vi "Flancos_2.vi"() -> ()   [LabVIEW 2017]
panel:
  out "Conteo 4":bool
  out "Conteo 3":bool
  out "Conteo 2":bool
  in  "Alarma":bool
  in  "Alarma 2":bool
  in  "Alarma 3":bool
  in  "Alarma 4":bool
  out "Conteo":bool
  in  "Seleccion":bool
  out "Waveform Chart":dbl(graph)
  out "Falling 4":dbl
  out "Rise 4":dbl
  out "Falling 3":dbl
  out "Rise 3":dbl
  out "Falling 2":dbl
  out "Rise 2":dbl
  out "Falling":dbl
  out "Rise":dbl
  in  "stop":bool
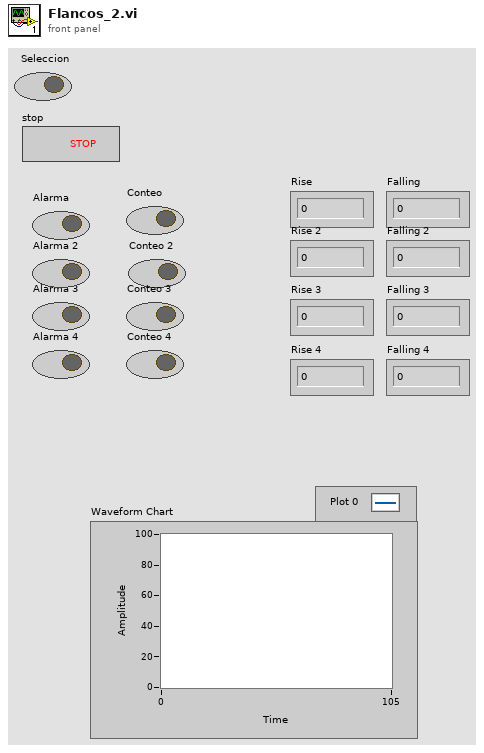
[diagram p1: front panel]
types:
  T1 = cluster{"Cont":i32, "Cont2":i32, "Cont3":i32, "Cont4":i32, "Bajada":i32, "Bajada 2":i32, "Bajada 3":i32, "Bajada 4":i32}
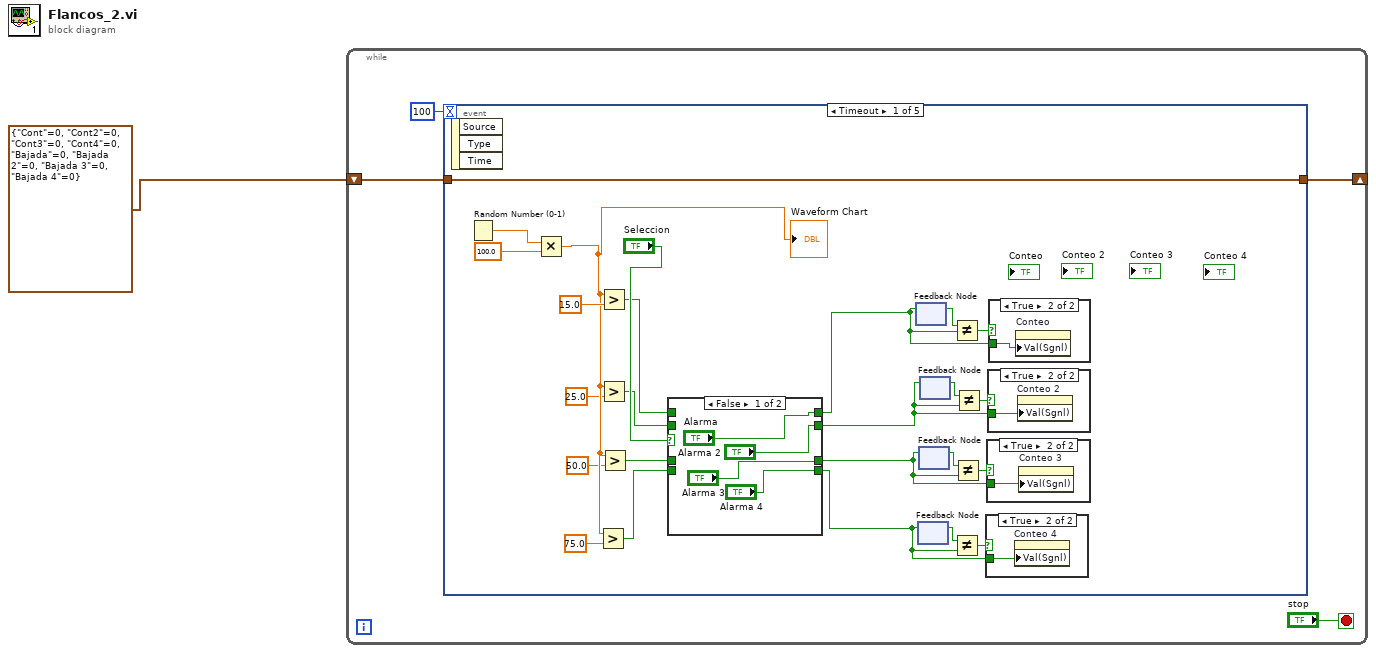
[diagram p0: block diagram]
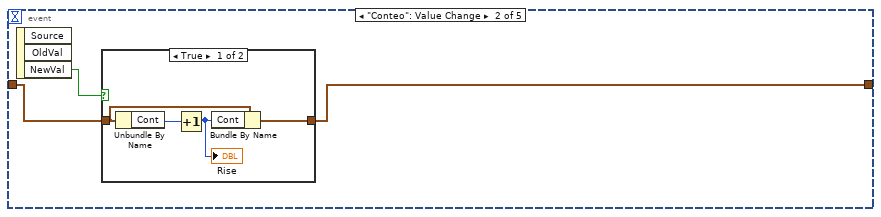
[diagram p7: hidden frame]
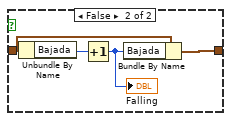
[diagram p8: hidden frame]
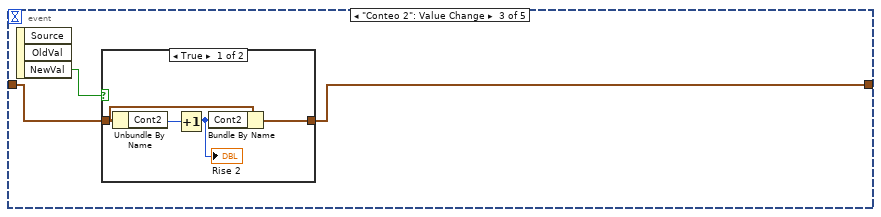
[diagram p9: hidden frame]
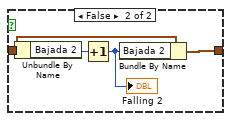
[diagram p10: hidden frame]
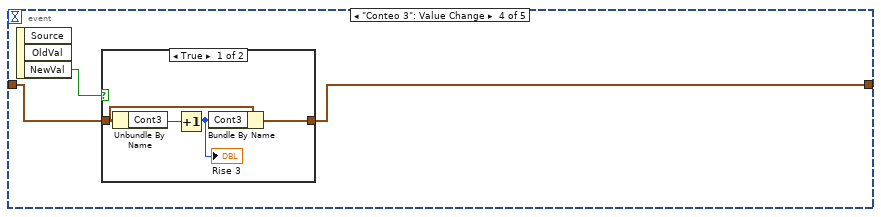
[diagram p11: hidden frame]
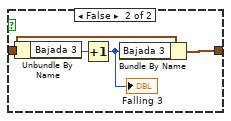
[diagram p12: hidden frame]
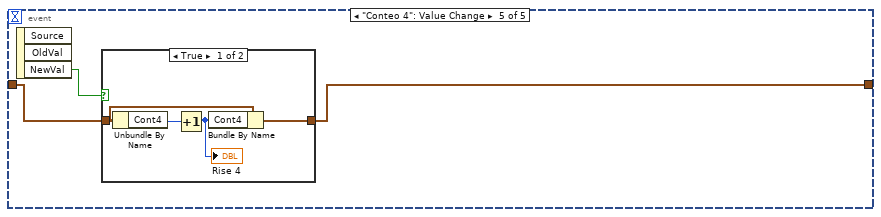
[diagram p13: hidden frame]
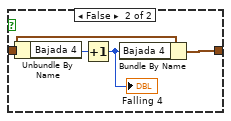
[diagram p14: hidden frame]
diagram:
  n1 = while {
    shift-right: [w3] -> _
    shift-left: T1 {"Cont"=0, "Cont2"=0, "Cont3"=0, "Cont4"=0, "Bajada"=0, "Bajada 2"=0, "Bajada 3"=0, "Bajada 4"=0} -> [w5]
    stop <- "stop" stop-if-true
    n2 = event shown="[0] Timeout" {
      selector: _ -> [_ _ _ _ _]
      dyn-events: _ -> [_ _ _ _ _]
      timeout: 100 -> [_ _ _ _ _]
      tunnel: w5 -> [w30 w45 w56 w67 w78]
      tunnel: [w30 w44 w55 w66 w77] -> w3
      event Timeout {
        n3 = event-data() -> ()  [unwired: 1 in, 3 out]
        n4 = Random Number (0-1)() -> (number: 0 to 1=w29:dbl)
        n5 = Multiply(x=w29, y=100.0) -> (x*y=w24:dbl)
        "Waveform Chart" <- w24
        n6 = Greater?(x=w24, y=75.0) -> (0:w16:bool)
        n7 = Greater?(x=w24, y=15.0) -> (0:w19:bool)
        n8 = Greater?(x=w24, y=25.0) -> (0:w18:bool)
        n9 = Greater?(x=w24, y=50.0) -> (0:w17:bool)
        n10 = case shown="False" "Seleccion" {
          tunnel: w19 -> [_ w41]
          tunnel: w18 -> [_ w40]
          tunnel: w17 -> [_ w39]
          tunnel: w16 -> [_ w38]
          tunnel: ["Alarma" w41] -> w15
          tunnel: ["Alarma 2" w40] -> w12
          tunnel: ["Alarma 3" w39] -> w9
          tunnel: ["Alarma 4" w38] -> w6
          frame False {
          }
          frame True {
          }
        }
        n11 = feedback #1() -> (w26:bool)  [unwired: 1 in]
        n12 = feedback-in #1(w15) -> ()
        n13 = feedback #2() -> (w8:bool)  [unwired: 1 in]
        n14 = feedback-in #2(w6) -> ()
        n15 = feedback #3() -> (w11:bool)  [unwired: 1 in]
        n16 = feedback-in #3(w9) -> ()
        n17 = feedback #4() -> (w14:bool)  [unwired: 1 in]
        n18 = feedback-in #4(w12) -> ()
        n19 = Not Equal?(x=w26, y=w15) -> (x != y?=w25:bool)
        n20 = Not Equal?(x=w8, y=w6) -> (x != y?=w7:bool)
        n21 = Not Equal?(x=w11, y=w9) -> (x != y?=w10:bool)
        n22 = Not Equal?(x=w14, y=w12) -> (x != y?=w13:bool)
        n23 = case shown="True" w7 {
          tunnel: w6 -> [_ w31]
          frame False {
          }
          frame True {
            n24 = property on="Conteo 4" class="Bool (strict)"("Val(Sgnl)"=w31) -> ()  [unwired: 2 in, 2 out]
          }
        }
        n25 = case shown="True" w10 {
          tunnel: w9 -> [_ w32]
          frame False {
          }
          frame True {
            n26 = property on="Conteo 3" class="Bool (strict)"("Val(Sgnl)"=w32) -> ()  [unwired: 2 in, 2 out]
          }
        }
        n27 = case shown="True" w13 {
          tunnel: w12 -> [_ w33]
          frame False {
          }
          frame True {
            n28 = property on="Conteo 2" class="Bool (strict)"("Val(Sgnl)"=w33) -> ()  [unwired: 2 in, 2 out]
          }
        }
        n29 = case shown="True" w25 {
          tunnel: w15 -> [_ w42]
          frame False {
          }
          frame True {
            n30 = property on="Conteo" class="Bool (strict)"("Val(Sgnl)"=w42) -> ()  [unwired: 2 in, 2 out]
          }
        }
      }
      event "Conteo": Value Change {
        n31 = event-data() -> ("NewVal"=w43:bool)  [unwired: 1 in, 2 out]
        n32 = case shown="True" w43 {
          tunnel: w45 -> [w48 w52]
          tunnel: [w47 w51] -> w44
          frame True {
            n33 = Unbundle By Name(w48) -> ("Cont"=w49:i32)
            n34 = Increment(x=w49) -> (x+1=w46:i32)
            "Rise" <- w46
            n35 = Bundle By Name(cluster=w48, "Cont"=w46) -> (w47:T1)
          }
          frame False {
            n36 = Unbundle By Name(w52) -> ("Bajada"=w53:i32)
            n37 = Increment(x=w53) -> (x+1=w50:i32)
            "Falling" <- w50
            n38 = Bundle By Name(cluster=w52, "Bajada"=w50) -> (w51:T1)
          }
        }
      }
      event "Conteo 2": Value Change {
        n39 = event-data() -> ("NewVal"=w54:bool)  [unwired: 1 in, 2 out]
        n40 = case shown="True" w54 {
          tunnel: w56 -> [w59 w63]
          tunnel: [w58 w62] -> w55
          frame True {
            n41 = Unbundle By Name(w59) -> ("Cont2"=w60:i32)
            n42 = Increment(x=w60) -> (x+1=w57:i32)
            "Rise 2" <- w57
            n43 = Bundle By Name(cluster=w59, "Cont2"=w57) -> (w58:T1)
          }
          frame False {
            n44 = Unbundle By Name(w63) -> ("Bajada 2"=w64:i32)
            n45 = Increment(x=w64) -> (x+1=w61:i32)
            "Falling 2" <- w61
            n46 = Bundle By Name(cluster=w63, "Bajada 2"=w61) -> (w62:T1)
          }
        }
      }
      event "Conteo 3": Value Change {
        n47 = event-data() -> ("NewVal"=w65:bool)  [unwired: 1 in, 2 out]
        n48 = case shown="True" w65 {
          tunnel: w67 -> [w70 w74]
          tunnel: [w69 w73] -> w66
          frame True {
            n49 = Unbundle By Name(w70) -> ("Cont3"=w71:i32)
            n50 = Increment(x=w71) -> (x+1=w68:i32)
            "Rise 3" <- w68
            n51 = Bundle By Name(cluster=w70, "Cont3"=w68) -> (w69:T1)
          }
          frame False {
            n52 = Unbundle By Name(w74) -> ("Bajada 3"=w75:i32)
            n53 = Increment(x=w75) -> (x+1=w72:i32)
            "Falling 3" <- w72
            n54 = Bundle By Name(cluster=w74, "Bajada 3"=w72) -> (w73:T1)
          }
        }
      }
      event "Conteo 4": Value Change {
        n55 = event-data() -> ("NewVal"=w76:bool)  [unwired: 1 in, 2 out]
        n56 = case shown="True" w76 {
          tunnel: w78 -> [w81 w85]
          tunnel: [w80 w84] -> w77
          frame True {
            n57 = Unbundle By Name(w81) -> ("Cont4"=w82:i32)
            n58 = Increment(x=w82) -> (x+1=w79:i32)
            "Rise 4" <- w79
            n59 = Bundle By Name(cluster=w81, "Cont4"=w79) -> (w80:T1)
          }
          frame False {
            n60 = Unbundle By Name(w85) -> ("Bajada 4"=w86:i32)
            n61 = Increment(x=w86) -> (x+1=w83:i32)
            "Falling 4" <- w83
            n62 = Bundle By Name(cluster=w85, "Bajada 4"=w83) -> (w84:T1)
          }
        }
      }
    }
  }
